vi "FlatToRichcif_manager_QueryErrorsResponse.vi"(5 "OutputClusterType":T1, 11 "InputCluster":T4) -> (3 "OutputCluster":T1)   [LabVIEW 2021, in "CIF_Manager_client.lvlib"]
uses:
  CIF_Manager_client.lvlib
  cif_manager_QueryErrorsResponse_Flat.ctl
  cif_manager_ErrorInfoList_Flat.ctl
  cif_manager_ErrorInfo_Flat.ctl
  cif_manager_QueryErrorsResponse.ctl
  cif_manager_ErrorInfoList.ctl
  cif_manager_ErrorInfo.ctl
  FlatToRichcif_manager_ErrorInfo.vi
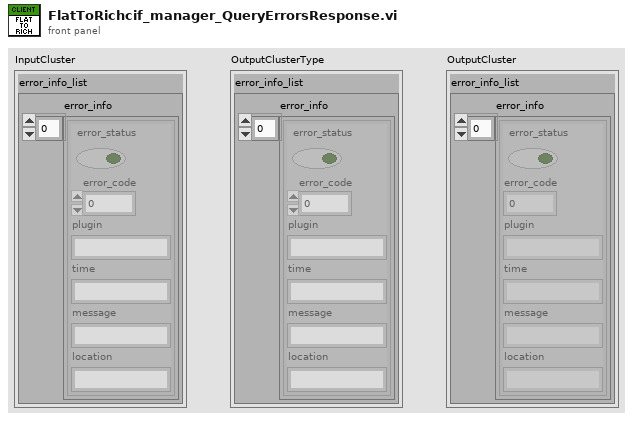
[diagram p1: front panel]
types:
  T1 = typedef "CIF_Manager_client.lvlib/cif_manager_QueryErrorsResponse.ctl" = cluster{"error_info_list":T2}
  T2 = typedef "CIF_Manager_client.lvlib/cif_manager_ErrorInfoList.ctl" = cluster{"error_info":T3[]}
  T3 = typedef "CIF_Manager_client.lvlib/cif_manager_ErrorInfo.ctl" = cluster{"error_status":bool, "error_code":i32, "plugin":string, "time":string, "message":string, "location":string}
  T4 = typedef "CIF_Manager_client.lvlib/cif_manager_QueryErrorsResponse_Flat.ctl" = cluster{"error_info_list":T5}
  T5 = typedef "CIF_Manager_client.lvlib/cif_manager_ErrorInfoList_Flat.ctl" = cluster{"error_info":T6[]}
  T6 = typedef "CIF_Manager_client.lvlib/cif_manager_ErrorInfo_Flat.ctl" = cluster{"error_status":bool, "error_code":i32, "plugin":string, "time":string, "message":string, "location":string}
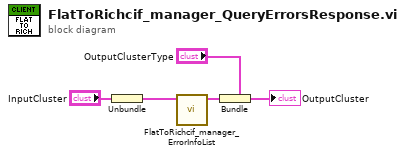
[diagram p0: block diagram]
diagram:
  n1 = Unbundle "Unbundle"("InputCluster") -> ("error_info_list"=w2:T5)
  n2 = call "FlatToRichcif_manager_ErrorInfoList.vi"("InputCluster"=w2) -> ("OutputCluster"=w1:T2)  [unwired: 10 in]
  n3 = Bundle "Bundle"(cluster="OutputClusterType", "error_info_list"=w1) -> (→"OutputCluster":T1)
